vi "诊断标定3 - 副本.vi"(8 "CAN端口":u16(ring), 9 "设备索引号":u16(ring), 10 "CAN卡类型":u32(ring)=21) -> ()   [LabVIEW 2013] (continued)
                n3216 = Index Array(array=w4254, index=w4244) -> (element=w4249:dbl)
                n3217 = Index Array(array=w4248, index=w4244) -> (element=w4246:string)
                n3218 = Index Array(array=w4251, index=w4244) -> (element=w4247:u32)
                n3219 = stacked-sequence {
                  seq-local: [_ _ _ w4278 _ _] -> [_ _ _ _ w4287 _]
                  tunnel: w4250 -> [_ _ w4266 _ _ _]
                  tunnel: w4249 -> [_ _ w4265 _ _ _]
                  tunnel: w4253 -> [_ _ w4260 _ _ _]
                  tunnel: w4252 -> [_ _ w4263 _ _ _]
                  tunnel: w4247 -> [_ _ w4261 _ _ _]
                  tunnel: w4246 -> [_ _ w4259 _ w4286 _]
                  tunnel: w4245 -> [_ _ _ _ _ w4299]
                  tunnel: w4244 -> [_ _ _ _ _ w4298]
                  tunnel: w4243 -> [_ _ _ _ _ w4296]
                  frame #0 {
                    w4257 = FALSE ("流控帧")
                    w4256 = TRUE ("流控帧 2")
                    n3220 = call <vilib>:"Set Busy.vi"("disable click? (T)"=w4257) -> ()  [unwired: 3 in, 8 out]
                    n3221 = global write "EV05全局变量1.vi" "读取超时"(w4257) -> ()
                    n3222 = global write "EV05全局变量1.vi" "流控帧"(w4257) -> ()
                    n3223 = local write "消除"(w4256) -> ()
                    n3224 = local write "控制1"(w4256) -> ()
                    n3225 = global write "EV05全局变量1.vi" "流控帧 2"(w4256) -> ()
                    n3226 = local write "写?"(w4256) -> ()
                  }
                  frame #1 {
                    n3227 = Wait Until Next ms Multiple(millisecond multiple=u32 50 ("毫秒倍数")) -> ()  [unwired: 1 out]
                  }
                  frame #2 {
                    n3228 = global write "全局 1.vi" "名称"(w4259) -> ()
                    n3229 = local write "命令序号"(w4261) -> ()
                    n3230 = local write "命令"(w4260) -> ()
                    n3231 = local read "设备索引号"() -> (w4268:u16)
                    n3232 = local read "CAN卡类型"() -> (w4269:u32)
                    n3233 = Increment(x=w4265) -> (x+1=w4262:dbl)
                    n3234 = local read "CAN端口"() -> (w4267:u16)
                    n3235 = Reshape Array(w4266, w4262) -> (w4264:dbl[])
                    n3236 = stacked-sequence {
                      tunnel: w4269 -> [_ w4277]
                      tunnel: w4268 -> [_ w4276]
                      tunnel: w4267 -> [_ w4275]
                      tunnel: w4264 -> [_ w4274]
                      tunnel: w4263 -> [_ w4273]
                      tunnel: w4261 -> [_ w4272]
                      tunnel: w4260 -> [_ w4271]
                      frame #0 {
                      }
                      frame #1 {
                        n3237 = call "多帧发送机制(EV05).vi"("can卡类型"=w4277, "设备索引号"=w4276, "CAN端口"=w4275, "命令"=w4271, "板号"=w4273, "命令序号"=w4272, "输入数据"=w4274) -> ("错误输出"=w4270:errorcluster)  [unwired: 1 in, 11 out]
                        n3238 = call <vilib>:"Clear Errors.vi"("error in (no error)"=w4270) -> ()  [unwired: 6 in, 1 out]
                      }
                    }
                  }
                  frame #3 {
                    n3239 = while {
                      tunnel: [w4280] -> w4278
                      i -> [w4285]
                      stop <- w4282 stop-if-true
                      n3240 = local read "强制终止读写标记"() -> (w4279:bool)
                      n3241 = global read "EV05全局变量1.vi" "读取超时"() -> (w4280:bool)
                      n3242 = Greater Or Equal?(x=w4285, y=30) -> (x >= y?=w4283:bool)
                      n3243 = Wait Until Next ms Multiple(millisecond multiple=u32 100 ("毫秒倍数")) -> ()  [unwired: 1 out]
                      n3244 = Compound Arithmetic op=OR(w4279, w4280, w4283) -> (w4282:bool)
                    }
                  }
                  frame #4 {
                    n3245 = call <vilib>:"Unset Busy.vi"() -> ()  [unwired: 2 in, 10 out]
                    n3246 = case shown="假" w4287 {
                      tunnel: w4286 -> [w4288 _]
                      frame False {
                        n3247 = control-ref of="结果"() -> (w4292:refnum<vi>)
                        n3248 = Concatenate Strings(w4288, "       写入失败" ("字符串")) -> (w4291:string)
                        n3249 = Build Array(w4291) -> (w4290:string[])
                        n3250 = call "表格编辑.vi"("新元素/子数组"=w4290, "活动单元格:单元格背景色"=u32 16740749, "MCListbox引用句柄"=w4292) -> ()  [unwired: 9 out]
                      }
                      frame True {
                      }
                    }
                  }
                  frame #5 {
                    n3251 = Increment(x=w4298) -> (x+1=w4294:i32)
                    n3252 = Equal?(x=w4299, y=w4294) -> (x = y?=w4297:bool)
                    n3253 = And(x=w4296, y=w4297) -> (x .and. y?=w4295:bool)
                    n3254 = case shown="真" w4295 {
                      frame False {
                      }
                      frame True {
                        n3255 = control-ref of="结果"() -> (w4303:refnum<vi>)
                        n3256 = Concatenate Strings("写入完成" ("字符串")) -> (w4302:string)
                        n3257 = Build Array(w4302) -> (w4301:string[])
                        n3258 = call "表格编辑.vi"("新元素/子数组"=w4301, "活动单元格:单元格背景色"=u32 21937, "MCListbox引用句柄"=w4303) -> ()  [unwired: 9 out]
                      }
                    }
                  }
                }
              }
              n3259 = local read "强制终止读写标记"() -> (w4196:bool)
              n3260 = Or(x=w4194, y=w4196) -> (x .or. y?=w4195:bool)
            }
            n3261 = stacked-sequence {
              tunnel: w4186 -> [_]
              frame #0 {
                n3262 = call <vilib>:"Unset Busy.vi"() -> ()  [unwired: 2 in, 10 out]
                n3263 = local write "强制终止读写标记"(FALSE ("强制停止")) -> ()
              }
            }
          }
          frame "单个读取" {
            n3264 = stacked-sequence {
              tunnel: [w4336] -> w4334
              frame #0 {
                n3265 = local read "主从选择"() -> (w4337:enum32{"主板", "从板"})
                n3266 = case shown="\"主板\", 默认" w4337 {
                  tunnel: [w4350 w4433] -> w4339
                  tunnel: [w4349 w4434] -> w4344
                  tunnel: [0 ("从板号") w4430] -> w4343
                  tunnel: [0 ("板号") u8 0 ("板号")] -> w4342
                  tunnel: [w4345 w4429] -> w4340
                  frame "主板", Default {
                    n3267 = local read "主板选项"() -> (w4346:string)
                    n3268 = case shown="\"二维码\"" w4346 {
                      tunnel: [_ u8[] [1, 2, 3, 4, 5, 6, 13, 8, 7, 9, 10, 11, 12] u8[] [1] u8[] [1] u8[] [1] u8[] [2] u8[] [3] u8[] [4] u8[] [5] u8[] [6] u8[] [13] u8[] [7] u8[] [8] u8[] [9] u8[] [10] u8[] [14] u8[] [11] u8[] [12] u8[] [2] u8[] [3] u8[] [1] u8[] [2] u8[] [1] u8[] [2] u8[] [3] u8[] [4] u8[] [1, 2, 3, 4]] -> w4350
                      tunnel: [_ u8 128 ("命令") u8 129 ("命令") u8 128 ("命令") u8 140 ("命令") u8 128 ("命令") u8 128 ("命令") u8 128 ("命令") u8 128 ("命令") u8 128 ("命令") u8 128 ("命令") u8 128 ("命令") u8 128 ("命令") u8 128 ("命令") u8 128 ("命令") u8 128 ("命令") u8 128 ("命令") u8 128 ("命令") u8 129 ("命令") u8 129 ("命令") u8 130 ("命令") u8 130 ("命令") u8 132 ("命令") u8 132 ("命令") u8 132 ("命令") u8 132 ("命令") u8 132 ("命令")] -> w4349
                      tunnel: [_ string[] ["产品编号", "电压个数", "通道电压数", "电压起始值", "温度个数", "温度起始值", "保险位置", "电池额定实际容量", "SOC", "配置文件版本", "参数修改记录", "车牌号", "SOH"] string[] ["一级故障阀值"] string[] ["产品编号"] string[] ["读二维码"] string[] ["电压个数"] string[] ["通道电压数"] string[] ["电压起始值"] string[] ["温度个数"] string[] ["温度起始值"] string[] ["保险位置"] string[] ["SOC"] string[] ["电池额定实际容量"] string[] ["配置文件版本"] string[] ["参数修改记录"] string[] ["校正时钟"] string[] ["车牌号"] string[] ["SOH"] string[] ["二级故障阀值"] string[] ["三级故障阀值"] string[] ["加热控制参数"] string[] ["充电控制参数"] string[] ["电池信息1"] string[] ["电池包组号"] string[] ["充放电安时"] string[] ["电池充放电次数"] string[] ["电池信息1", "电池包组号", "充放电安时", "电池充放电次数"]] -> w4345
                      frame "假", Default {
                      }
                      frame "项目信息" {
                      }
                      frame "SOC过低", "SOC过高", "SOH过低", "充电电流过高", "单体电压过低", "单体电压过高", "单组电压不均衡", "单组温度不均衡", "放电电流过高", "极柱温度过高", "内阻过大", "温度过低", "温度过高", "一级故障阀值", "整组电压不均衡", "整组温度不均衡", "总电压过低", "总电压过高" {
                      }
                      frame "产品编号" {
                      }
                      frame "二维码" {
                      }
                      frame "电压个数" {
                      }
                      frame "通道电压数" {
                      }
                      frame "电压起始值" {
                      }
                      frame "温度个数" {
                      }
                      frame "温度起始值" {
                      }
                      frame "保险位置" {
                      }
                      frame "SOC" {
                      }
                      frame "电池额定实际容量" {
                      }
                      frame "配置文件版本" {
                      }
                      frame "参数修改记录" {
                      }
                      frame "校正时钟" {
                      }
                      frame "车牌号" {
                      }
                      frame "SOH" {
                      }
                      frame "SOC过低(2)", "SOC过高(2)", "SOH过低(2)", "充电电流过高(2)", "单体电压过低(2)", "单体电压过高(2)", "单组电压不均衡(2)", "单组温度不均衡(2)", "二级故障阀值", "放电电流过高(2)", "极柱温度过高(2)", "内阻过大(2)", "温度过低(2)", "温度过高(2)", "整组电压不均衡(2)", "整组温度不均衡(2)", "总电压过低(2)", "总电压过高(2)" {
                      }
                      frame "SOC过低(3)", "SOC过高(3)", "SOH过低(3)", "充电电流过高(3)", "单体电压过低(3)", "单体电压过高(3)", "单组电压不均衡(3)", "单组温度不均衡(3)", "放电电流过高(3)", "极柱温度过高(3)", "内阻过大(3)", "三级故障阀值", "温度过低(3)", "温度过高(3)", "整组电压不均衡(3)", "整组温度不均衡(3)", "总电压过低(3)", "总电压过高(3)" {
                      }
                      frame "风机关闭温差", "风机关闭温度", "风机开启温差", "风机开启温度", "加热关闭温差", "加热关闭温度", "加热开启温度", "加热控制参数" {
                      }
                      frame "充电控制参数", "电流步长", "最大允许充电电流", "最大允许充电温度", "最大允许单体电压", "最大允许总电压", "最小允许充电电流", "最小允许充电温度", "最小允许单体电压" {
                      }
                      frame "电池信息1" {
                      }
                      frame "电池包组号" {
                      }
                      frame "充放电安时" {
                      }
                      frame "电池充放电次数" {
                      }
                      frame "电池信息" {
                      }
                    }
                  }
                  frame "从板" {
                    n3269 = local read "从板选项"() -> (w4431:string)
                    n3270 = case shown="\"二维码\"" w4431 {
                      tunnel: [_ u8 0 ("命令") u8 10 ("命令") u8 0 ("命令") u8 0 ("命令") u8 0 ("命令") u8 0 ("命令") u8 0 ("命令") u8 0 ("命令") u8 2 ("命令") u8 2 ("命令") u8 2 ("命令") u8 3 ("命令") u8 6 ("命令") u8 6 ("命令") u8 6 ("命令") u8 3 ("命令") u8 3 ("命令") u8 3 ("命令") u8 3 ("命令") u8 3 ("命令") u8 3 ("命令") u8 3 ("命令")] -> w4434
                      tunnel: [_ u8[] [6] u8[] [1] u8[] [6, 1, 2, 3, 4, 5] u8[] [1] u8[] [2] u8[] [3] u8[] [4] u8[] [5] u8[] [1] u8[] [2] u8[] [3] u8[] [1, 2, 3, 4, 5, 6, 7] u8[] [1, 2] u8[] [2] u8[] [1] u8[] [1] u8[] [2] u8[] [3] u8[] [4] u8[] [5] u8[] [6] u8[] [7]] -> w4433
                      tunnel: [_ string[] ["从板号"] string[] ["读二维码"] string[] ["从板号", "电压起始值", "通道电压个数", "保险位置", "温度起始值", "加热控制参数"] string[] ["电压起始值"] string[] ["通道电压节数"] string[] ["保险位置"] string[] ["温度起始值"] string[] ["加热控制参数"] string[] ["一级故障阀值"] string[] ["二级故障阀值"] string[] ["三级故障阀值"] string[] ["电池包信息1", "电池包序号", "充放电安时", "充电次数时间", "SOC", "车牌号", "充电参数"] string[] ["均衡阀值", "充电结束电压"] string[] ["充电结束电压"] string[] ["均衡阀值"] string[] ["电池包信息1"] string[] ["电池包序号"] string[] ["充放电安时"] string[] ["充电次数时间"] string[] ["SOC"] string[] ["车牌号"] string[] ["充电参数"]] -> w4429
                      frame "假", Default {
                      }
                      frame "从板号" {
                      }
                      frame "二维码" {
                      }
                      frame "从板信息" {
                      }
                      frame "电压个数" {
                      }
                      frame "通道电压节数" {
                      }
                      frame "保险位置" {
                      }
                      frame "温度个数" {
                      }
                      frame "风机关闭温差", "风机关闭温度", "风机开启温差", "风机开启温度", "加热关闭温差", "加热关闭温度", "加热开启温度", "加热控制参数" {
                      }
                      frame "SOC过低", "电压不均衡", "电压过低", "电压过高", "温度不均衡", "温度过低", "温度过高", "一级故障阀值" {
                      }
                      frame "SOC过低(2)", "电压不均衡(2)", "电压过低(2)", "电压过高(2)", "二级故障阀值", "温度不均衡(2)", "温度过低(2)", "温度过高(2)" {
                      }
                      frame "SOC过低(3)", "电压不均衡(3)", "电压过低(3)", "电压过高(3)", "三级故障阀值", "温度不均衡(3)", "温度过低(3)", "温度过高(3)" {
                      }
                      frame "快换参数" {
                      }
                      frame "均衡参数" {
                      }
                      frame "充电结束电压" {
                      }
                      frame "均衡阀值" {
                      }
                      frame "电池包信息1" {
                      }
                      frame "电池包序号" {
                      }
                      frame "充放电安时" {
                      }
                      frame "充电次数时间" {
                      }
                      frame "SOC" {
                      }
                      frame "车牌号" {
                      }
                      frame "充电参数" {
                      }
                    }
                    n3271 = local read "从板号"() -> (w4430:u8)
                  }
                }
                n3272 = Build Array(w4342) -> (w4341:i32[])
                n3273 = local write "命令"(w4344) -> ()
                n3274 = Array Size(array=w4339) -> (size(s)=w4338:i32)
                n3275 = for {
                  tunnel: w4339 -> [w4509] mode=indexing
                  tunnel: w4344 -> [w4508]
                  tunnel: w4343 -> [w4507]
                  tunnel: w4341 -> [w4506]
                  tunnel: w4340 -> [w4505] mode=indexing
                  tunnel: w4338 -> [w4504]
                  tunnel: w4337 -> [w4502]
                  tunnel: [w4501] -> w4336
                  i -> [w4503]
                  n3276 = while {
                    tunnel: w4509 -> [w4518]
                    tunnel: w4508 -> [w4517]
                    tunnel: w4507 -> [w4516]
                    tunnel: w4506 -> [w4515]
                    tunnel: w4505 -> [w4514]
                    tunnel: w4504 -> [w4513]
                    tunnel: w4503 -> [w4512]
                    tunnel: w4502 -> [w4511]
                    tunnel: [w4510] -> w4501
                    stop <- w4510 stop-if-true
                    n3277 = stacked-sequence {
                      seq-local: [_ _ _ _ w4668 _ _] -> [_ _ _ _ _ w4677 _]
                      tunnel: w4518 -> [_ _ _ w4656 _ _ _]
                      tunnel: w4517 -> [_ _ _ w4655 _ _ _]
                      tunnel: w4516 -> [_ _ _ w4654 _ _ _]
                      tunnel: w4515 -> [_ _ _ w4653 _ _ _]
                      tunnel: [_ _ _ _ w4669 _ _] -> w4510
                      tunnel: w4514 -> [w4520 _ _ _ _ w4678 _]
                      tunnel: w4513 -> [_ _ _ _ _ _ w4688]
                      tunnel: w4512 -> [_ _ _ _ _ _ w4687]
                      tunnel: w4511 -> [w4519 _ _ _ _ _ _]
                      frame #0 {
                        n3278 = case shown="\"从板\"" w4519 {
                          tunnel: w4520 -> [w4521 w4613]
                          frame "主板", Default {
                            n3279 = case shown="\"读二维码\"" w4521 {
                              frame "假", Default {
                              }
                              frame "产品编号" {
                                n3280 = control-ref of="产品编号"() -> (w4523:refnum<vi>)
                                n3281 = property class="Str"(reference=w4523, "Value"="") -> ()  [unwired: 1 in, 2 out]
                              }
                              frame "读二维码" {
                                n3282 = local write "二维码信息"("" ("二维码信息")) -> ()
                              }
                              frame "电压个数" {
                                n3283 = local read "从板个数"() -> (w4525:dbl)
                                n3284 = control-ref of="项目信息"() -> (w4529:refnum<vi>)
                                n3285 = for {
                                N: w4525 -> [_]
                                tunnel: [""] -> w4528 mode=indexing
                                }
                                n3286 = call "表格数据输入-8.6.vi"("行数"=u32 0, "列数"=u32 1, "字符串数组"=w4528, "表格引用"=w4529) -> ()  [unwired: 8 in]
                              }
                              frame "通道电压数" {
                                n3287 = control-ref of="项目信息"() -> (w4535:refnum<vi>)
                                n3288 = for {
                                N: 20 -> [_]
                                tunnel: [""] -> w4534 mode=indexing
                                }
                                n3289 = local read "从板个数"() -> (w4536:dbl)
                                n3290 = Increment(x=w4536) -> (x+1=w4532:dbl)
                                n3291 = call "表格数据输入-8.6.vi"("行数"=w4532, "列数"=u32 1, "字符串数组"=w4534, "表格引用"=w4535) -> ()  [unwired: 8 in]
                              }
                              frame "电压起始值" {
                                n3292 = local read "从板个数"() -> (w4540:dbl)
                                n3293 = Increment(x=w4540) -> (x+1=w4539:dbl)
                                n3294 = control-ref of="项目信息"() -> (w4546:refnum<vi>)
                                n3295 = for {
                                N: w4539 -> [_]
                                tunnel: [""] -> w4545 mode=indexing
                                }
                                n3296 = Multiply(x=u8 1, y=w4540) -> (x*y=w4542:dbl)
                                n3297 = Add(x=w4542, y=u8 21) -> (x+y=w4538:dbl)
                                n3298 = call "表格数据输入-8.6.vi"("行数"=w4538, "列数"=u32 1, "字符串数组"=w4545, "表格引用"=w4546) -> ()  [unwired: 8 in]
                              }
                              frame "温度个数" {
                                n3299 = local read "从板个数"() -> (w4550:dbl)
                                n3300 = Increment(x=w4550) -> (x+1=w4549:dbl)
                                n3301 = control-ref of="项目信息"() -> (w4556:refnum<vi>)
                                n3302 = for {
                                N: w4549 -> [_]
                                tunnel: [""] -> w4555 mode=indexing
                                }
                                n3303 = Multiply(x=u8 2, y=w4550) -> (x*y=w4552:dbl)
                                n3304 = Add(x=w4552, y=u8 22) -> (x+y=w4548:dbl)
                                n3305 = call "表格数据输入-8.6.vi"("行数"=w4548, "列数"=u32 1, "字符串数组"=w4555, "表格引用"=w4556) -> ()  [unwired: 8 in]
                              }
                              frame "温度起始值" {
                                n3306 = local read "从板个数"() -> (w4560:dbl)
                                n3307 = Increment(x=w4560) -> (x+1=w4559:dbl)
                                n3308 = control-ref of="项目信息"() -> (w4566:refnum<vi>)
                                n3309 = for {
                                N: w4559 -> [_]
                                tunnel: [""] -> w4565 mode=indexing
                                }
                                n3310 = Multiply(x=u8 3, y=w4560) -> (x*y=w4562:dbl)
                                n3311 = Add(x=w4562, y=u8 23) -> (x+y=w4558:dbl)
                                n3312 = call "表格数据输入-8.6.vi"("行数"=w4558, "列数"=u32 1, "字符串数组"=w4565, "表格引用"=w4566) -> ()  [unwired: 8 in]
                              }
                              frame "保险位置" {
                                n3313 = local read "从板个数"() -> (w4570:dbl)
                                n3314 = control-ref of="项目信息"() -> (w4576:refnum<vi>)
                                n3315 = for {
                                N: 10 -> [_]
                                tunnel: [""] -> w4575 mode=indexing
                                }
                                n3316 = Multiply(x=u8 4, y=w4570) -> (x*y=w4572:dbl)
                                n3317 = Add(x=w4572, y=u8 24) -> (x+y=w4569:dbl)
                                n3318 = call "表格数据输入-8.6.vi"("行数"=w4569, "列数"=u32 1, "字符串数组"=w4575, "表格引用"=w4576) -> ()  [unwired: 8 in]
                              }
                              frame "电池额定实际容量" {
                                w4578 = 0.0 ("值")
                                n3319 = control-ref of="电池实际容量(A)"() -> (w4579:refnum<vi>)
                                n3320 = control-ref of="电池额定容量(A)"() -> (w4580:refnum<vi>)
                                n3321 = property class="DigNum (严格)"(reference=w4579, "Value"=w4578) -> ()  [unwired: 1 in, 2 out]
                                n3322 = property class="DigNum (严格)"(reference=w4580, "Value"=w4578) -> ()  [unwired: 1 in, 2 out]
                              }
                              frame "SOC" {
                                n3323 = control-ref of="SOC(%)"() -> (w4581:refnum<vi>)
                                n3324 = property class="DigNum (严格)"(reference=w4581, "Value"=0.0 ("值")) -> ()  [unwired: 1 in, 2 out]
                              }
                              frame "配置文件版本" {
                                n3325 = control-ref of="配置文件版本"() -> (w4583:refnum<vi>)
                                n3326 = property class="Str"(reference=w4583, "Value"="" ("值")) -> ()  [unwired: 1 in, 2 out]
                              }
                              frame "参数修改记录" {
                                n3327 = control-ref of="使用者"() -> (w4586:refnum<vi>)
                                n3328 = control-ref of="系统时钟"() -> (w4587:refnum<vi>)
                                n3329 = property class="DigNum (严格)"(reference=w4586, "Value"=0.0 ("值")) -> ()  [unwired: 1 in, 2 out]
                                n3330 = property class="Str"(reference=w4587, "Value"="" ("值")) -> ()  [unwired: 1 in, 2 out]
                              }
                              frame "校正时钟" {
                                n3331 = control-ref of="系统时钟"() -> (w4589:refnum<vi>)
                                n3332 = property class="Str"(reference=w4589, "Value"="" ("值")) -> ()  [unwired: 1 in, 2 out]
                              }
                              frame "车牌号" {
                                n3333 = control-ref of="车架(牌)号"() -> (w4591:refnum<vi>)
                                n3334 = property class="Str"(reference=w4591, "Value"="" ("值")) -> ()  [unwired: 1 in, 2 out]
                              }
                              frame "SOH" {
                                n3335 = control-ref of="SOH(%)"() -> (w4594:refnum<vi>)
                                n3336 = property class="DigNum (严格)"(reference=w4594, "Value"=0.0 ("值")) -> ()  [unwired: 1 in, 2 out]
                              }
                              frame "一级故障阀值" {
                                n3337 = local write "一级故障"(T10 {"总电压过高"=0.0, "整组电压不均衡"=0.0, "SOC过高"=0.0, "单体电压过高"=0.0, "总电压过低"=0.0, "温度过高"=0.0, "温度过低"=0.0, "单组电压不均衡"=0.0, "整组温度不均衡"=0.0, "单组温度不均衡"=0.0, "单体电压过低"=0.0, "充电电流过高"=0.0, "放电电流过高"=0.0, "SOC过低"=0.0, "内阻过大"=0.0, "极柱温度过高"=0.0, "SOH过低"=0.0} ("一级故障")) -> ()
                              }
                              frame "二级故障阀值" {
                                n3338 = local write "一级故障 2"(T10 {"总电压过高"=0.0, "整组电压不均衡"=0.0, "SOC过高"=0.0, "单体电压过高"=0.0, "总电压过低"=0.0, "温度过高"=0.0, "温度过低"=0.0, "单组电压不均衡"=0.0, "整组温度不均衡"=0.0, "单组温度不均衡"=0.0, "单体电压过低"=0.0, "充电电流过高"=0.0, "放电电流过高"=0.0, "SOC过低"=0.0, "内阻过大"=0.0, "极柱温度过高"=0.0, "SOH过低"=0.0} ("一级故障")) -> ()
                              }
                              frame "三级故障阀值" {
                                n3339 = local write "一级故障 3"(T10 {"总电压过高"=0.0, "整组电压不均衡"=0.0, "SOC过高"=0.0, "单体电压过高"=0.0, "总电压过低"=0.0, "温度过高"=0.0, "温度过低"=0.0, "单组电压不均衡"=0.0, "整组温度不均衡"=0.0, "单组温度不均衡"=0.0, "单体电压过低"=0.0, "充电电流过高"=0.0, "放电电流过高"=0.0, "SOC过低"=0.0, "内阻过大"=0.0, "极柱温度过高"=0.0, "SOH过低"=0.0} ("一级故障")) -> ()
                              }
                              frame "加热控制参数" {
                                n3340 = local write "加热控制参数"(T11 {"风机开启温度"=0.0, "风机关闭温度"=0.0, "加热开启温度"=0.0, "加热关闭温度"=0.0, "风机开启温差"=0.0, "风机关闭温差"=0.0, "加热关闭温差"=0.0} ("加热控制参数")) -> ()
                              }
                              frame "充电控制参数" {
                                n3341 = local write "一级故障 5"(T12 {"最大允许单体电压"=0.0, "最大允许总电压"=0.0, "最小允许单体电压"=0.0, "最大允许充电电流"=0.0, "最小允许充电电流"=0.0, "最大允许充电温度"=0.0, "最小允许充电温度"=0.0, "电流步长"=0.0} ("一级故障 5")) -> ()
                              }
                              frame "电池信息1" {
                                w4600 = ""
                                w4601 = 0.0 ("电池串联")
                                n3342 = local read "电池信息"() -> (w4603:T13)
                                n3343 = Bundle By Name(cluster=w4603, "电池串联"=w4601, "电池并联"=w4601, "电池包额定容量"=w4601, "电池包额定能量(kWh)"=w4601, "电池包额定总电压"=w4601, "实际容量"=w4601, "电池厂家"=w4600, "电池类型"=w4600, "电池生产日期"=w4600) -> (w4602:T13)
                                n3344 = local write "电池信息"(w4602) -> ()
                              }
                              frame "电池包组号" {
                                n3345 = local read "电池信息"() -> (w4606:T13)
                                n3346 = Bundle By Name(cluster=w4606, "电池包组号"="") -> (w4605:T13)
                                n3347 = local write "电池信息"(w4605) -> ()
                              }
                              frame "充放电安时" {
                                w4607 = 0.0 ("累计充电总安时")
                                n3348 = local read "电池信息"() -> (w4609:T13)
                                n3349 = Bundle By Name(cluster=w4609, "累计充电总安时"=w4607, "累计放电总安时"=w4607) -> (w4608:T13)
                                n3350 = local write "电池信息"(w4608) -> ()
                              }
                              frame "电池充放电次数" {
                                w4610 = 0.0 ("累计充电总安时")
                                n3351 = local read "电池信息"() -> (w4612:T13)
                                n3352 = Bundle By Name(cluster=w4612, "电池充满次数"=w4610, "电池放空次数"=w4610, "电池充电次数"=w4610) -> (w4611:T13)
                                n3353 = local write "电池信息"(w4611) -> ()
                              }
                            }
                          }
                          frame "从板" {
                            n3354 = case shown="\"读二维码\"" w4613 {
                              frame "假", Default {
                              }
                              frame "电压起始值" {
                                n3355 = control-ref of="项目信息 2"() -> (w4615:refnum<vi>)
                                n3356 = for {
                                N: 1 -> [_]
                                tunnel: [""] -> w4618 mode=indexing
                                }
                                n3357 = call "表格数据输入-8.6.vi"("行数"=u32 0, "列数"=u32 1, "字符串数组"=w4618, "表格引用"=w4615) -> ()  [unwired: 8 in]
                              }
                              frame "读二维码" {
                                n3358 = local write "二维码信息 2"("" ("二维码信息 2")) -> ()
                              }
                              frame "通道电压节数" {
                                n3359 = control-ref of="项目信息 2"() -> (w4621:refnum<vi>)
                                n3360 = for {
                                N: 5 -> [_]
                                tunnel: [""] -> w4625 mode=indexing
                                }
                                n3361 = call "表格数据输入-8.6.vi"("行数"=u32 22, "列数"=u32 1, "字符串数组"=w4625, "表格引用"=w4621) -> ()  [unwired: 8 in]
                              }
                              frame "保险位置" {
                                n3362 = control-ref of="项目信息 2"() -> (w4627:refnum<vi>)
                                n3363 = for {
                                N: 20 -> [_]
                                tunnel: [""] -> w4631 mode=indexing
                                }
                                n3364 = call "表格数据输入-8.6.vi"("行数"=u32 2, "列数"=u32 1, "字符串数组"=w4631, "表格引用"=w4627) -> ()  [unwired: 8 in]
                              }
                              frame "温度起始值" {
                                n3365 = control-ref of="项目信息 2"() -> (w4633:refnum<vi>)
                                n3366 = for {
                                N: 1 -> [_]
                                tunnel: [""] -> w4637 mode=indexing
                                }
                                n3367 = call "表格数据输入-8.6.vi"("行数"=u32 1, "列数"=u32 1, "字符串数组"=w4637, "表格引用"=w4633) -> ()  [unwired: 8 in]
                              }
                              frame "加热控制参数" {
                                n3368 = local write "加热控制参数"(T11 {"风机开启温度"=0.0, "风机关闭温度"=0.0, "加热开启温度"=0.0, "加热关闭温度"=0.0, "风机开启温差"=0.0, "风机关闭温差"=0.0, "加热关闭温差"=0.0} ("加热控制参数")) -> ()
                              }
                              frame "一级故障阀值" {
                                n3369 = local write "一级故障 6"(T15 {"电压过高"=0.0, "电压过低"=0.0, "温度过高"=0.0, "温度过低"=0.0, "电压不均衡(V)"=0.0, "温度不均衡"=0.0, "SOC过低"=0.0} ("一级故障 6")) -> ()
                              }
                              frame "二级故障阀值" {
                                n3370 = local write "一级故障 7"(T15 {"电压过高"=0.0, "电压过低"=0.0, "温度过高"=0.0, "温度过低"=0.0, "电压不均衡(V)"=0.0, "温度不均衡"=0.0, "SOC过低"=0.0} ("一级故障 7")) -> ()
                              }
                              frame "三级故障阀值" {
                                n3371 = local write "一级故障 8"(T15 {"电压过高"=0.0, "电压过低"=0.0, "温度过高"=0.0, "温度过低"=0.0, "电压不均衡(V)"=0.0, "温度不均衡"=0.0, "SOC过低"=0.0} ("一级故障 7")) -> ()
                              }
                              frame "均衡参数" {
                                n3372 = local write "均衡参数"(T17 {"充电结束电压(90%)"=0.0, "充电结束电压(91%)"=0.0, "充电结束电压(92%)"=0.0, "充电结束电压(93%)"=0.0, "充电结束电压(94%)"=0.0, "均衡计算-电压高阀值1级"=0.0, "均衡计算-电压高阀值2级"=0.0, "均衡计算-电压低阀值1级"=0.0, "均衡计算-电压低阀值2级"=0.0, "均衡计算-最低电压阀值"=0.0, "均衡停止-最低电压阀值"=0.0, "均衡计算-电压极差阀值"=0.0, "充电结束电压(95%)"=0.0, "充电结束电压(96%)"=0.0, "充电结束电压(97%)"=0.0, "充电结束电压(98%)"=0.0, "充电结束电压(99%)"=0.0, "充电结束电压(100%)"=0.0} ("均衡参数")) -> ()
                              }
                              frame "均衡阀值" {
                                w4644 = sgl 0.0 ("均衡计算-电压高阀值1级")
                                n3373 = local read "均衡参数"() -> (w4645:T17)
                                n3374 = Bundle By Name(cluster=w4645, "均衡计算-电压高阀值1级"=w4644, "均衡计算-电压高阀值2级"=w4644, "均衡计算-电压低阀值1级"=w4644, "均衡计算-电压低阀值2级"=w4644, "均衡计算-最低电压阀值"=w4644, "均衡停止-最低电压阀值"=w4644, "均衡计算-电压极差阀值"=w4644) -> (w4646:T17)
                                n3375 = local write "均衡参数"(w4646) -> ()
                              }
                              frame "充电结束电压" {
                                w4647 = sgl 0.0 ("均衡计算-电压高阀值1级")
                                n3376 = local read "均衡参数"() -> (w4648:T17)
                                n3377 = Bundle By Name(cluster=w4648, "充电结束电压(90%)"=w4647, "充电结束电压(91%)"=w4647, "充电结束电压(92%)"=w4647, "充电结束电压(93%)"=w4647, "充电结束电压(94%)"=w4647, "充电结束电压(95%)"=w4647, "充电结束电压(96%)"=w4647, "充电结束电压(97%)"=w4647, "充电结束电压(98%)"=w4647, "充电结束电压(99%)"=w4647, "充电结束电压(100%)"=w4647) -> (w4649:T17)
                                n3378 = local write "均衡参数"(w4649) -> ()
                              }
                            }
                          }
                        }
                      }
                      frame #1 {
                        w4650 = FALSE ("流控帧")
                        w4651 = TRUE ("流控帧 2")
                        n3379 = global write "EV05全局变量1.vi" "写入超时"(w4650) -> ()
                        n3380 = global write "EV05全局变量1.vi" "流控帧"(w4650) -> ()
                        n3381 = local write "写?"(w4650) -> ()
                        n3382 = call <vilib>:"Set Busy.vi"("disable click? (T)"=w4650) -> ()  [unwired: 3 in, 8 out]
                        n3383 = local write "消除"(w4651) -> ()
                        n3384 = local write "控制1"(w4651) -> ()
                        n3385 = global write "EV05全局变量1.vi" "流控帧 2"(w4651) -> ()
                      }
                      frame #2 {
                        n3386 = Wait Until Next ms Multiple(millisecond multiple=u32 150 ("毫秒倍数")) -> ()  [unwired: 1 out]
                      }
                      frame #3 {
                        n3387 = local read "设备索引号"() -> (w4658:u16)
                        n3388 = local read "CAN卡类型"() -> (w4659:u32)
                        n3389 = local read "CAN端口"() -> (w4657:u16)
                        n3390 = stacked-sequence {
                          tunnel: w4659 -> [_ w4667]
                          tunnel: w4658 -> [_ w4666]
                          tunnel: w4657 -> [_ w4665]
                          tunnel: w4656 -> [_ w4664]
                          tunnel: w4655 -> [_ w4663]
                          tunnel: w4654 -> [_ w4662]
                          tunnel: w4653 -> [_ w4661]
                          frame #0 {
                          }
                          frame #1 {
                            n3391 = call "多帧发送机制(EV05).vi"("can卡类型"=w4667, "设备索引号"=w4666, "CAN端口"=w4665, "命令"=w4663, "板号"=w4662, "命令序号"=w4664, "输入数据"=w4661) -> ("错误输出"=w4660:errorcluster)  [unwired: 1 in, 11 out]
                            n3392 = call <vilib>:"Clear Errors.vi"("error in (no error)"=w4660) -> ()  [unwired: 6 in, 1 out]
                          }
                        }
                        "命令序号" <- w4656
                      }
                      frame #4 {
                        n3393 = while {
                          tunnel: [w4672] -> w4669
                          tunnel: [w4671] -> w4668
                          i -> [w4675]
                          stop <- w4672 stop-if-true
                          n3394 = local read "强制终止读写标记"() -> (w4670:bool)
                          n3395 = global read "EV05全局变量1.vi" "写入超时"() -> (w4671:bool)
                          n3396 = Greater Or Equal?(x=w4675, y=30) -> (x >= y?=w4673:bool)
                          n3397 = Compound Arithmetic op=OR(w4670, w4671, w4673) -> (w4672:bool)
                          n3398 = Wait Until Next ms Multiple(millisecond multiple=u32 100 ("毫秒倍数")) -> ()  [unwired: 1 out]
                        }
                      }
                      frame #5 {
                        n3399 = case shown="假" w4677 {
                          tunnel: w4678 -> [w4681 _]
                          frame False {
                            n3400 = control-ref of="结果"() -> (w4680:refnum<vi>)
                            n3401 = Concatenate Strings(w4681, "     读取失败" ("字符串")) -> (w4683:string)
                            n3402 = Build Array(w4683) -> (w4679:string[])
                            n3403 = call "表格编辑.vi"("新元素/子数组"=w4679, "活动单元格:单元格背景色"=u32 16740749, "MCListbox引用句柄"=w4680) -> ()  [unwired: 9 out]
                          }
                          frame True {
                          }
                        }
                      }
                      frame #6 {
                        n3404 = Increment(x=w4687) -> (x+1=w4686:i32)
                        n3405 = Equal?(x=w4688, y=w4686) -> (x = y?=w4685:bool)
                        n3406 = case shown="真" w4685 {
                          frame False {
                          }
                          frame True {
                            n3407 = control-ref of="结果"() -> (w4690:refnum<vi>)
                            n3408 = Concatenate Strings("读取完成" ("字符串")) -> (w4692:string)
                            n3409 = Build Array(w4692) -> (w4689:string[])
                            n3410 = call "表格编辑.vi"("新元素/子数组"=w4689, "活动单元格:单元格背景色"=u32 21937, "MCListbox引用句柄"=w4690) -> ()  [unwired: 9 out]
                          }
                        }
                      }
                    }
                  }
                }
              }
            }
            n3411 = stacked-sequence {
              tunnel: w4334 -> [_]
              frame #0 {
                n3412 = call <vilib>:"Unset Busy.vi"() -> ()  [unwired: 11 in, 1 out]
                n3413 = local write "强制终止读写标记"(FALSE ("强制停止")) -> ()
              }
            }
          }
          frame "全部读取" {
            n3414 = stacked-sequence {
              seq-local: [w4698 _ _] -> [_ _ w5259]
              seq-local: [w4697 _ _] -> [_ _ w5258]
              tunnel: [_ w4889 _] -> w4695
              frame #0 {
                n3415 = local read "主从选择"() -> (w4698:enum32{"主板", "从板"})
                n3416 = local read "路径"() -> (w4699:path)
                n3417 = Empty String/Path?(string/path=w4699) -> (empty?=w4697:bool)
                n3418 = disable-structure shown="禁用" {
                  disable-tunnel: w4699 -> [w4702 _]
                  disable-tunnel: w4697 -> [w4701 _]
                  disable-tunnel: w4698 -> [w4700 _]
                  frame Disabled {
                    n3419 = case shown="假" w4701 {
                      tunnel: w4702 -> [w4706 _]
                      tunnel: w4700 -> [w4705 _]
                      frame False {
                        n3420 = control-ref of="结果"() -> (w4703:refnum<vi>)
                        n3421 = call-poly <vilib>:"Read From Spreadsheet File.vi"("file path (dialog if empty)"=w4706) -> ("all rows"=w4704:string[][])  [unwired: 3 in, 7 out]
                        n3422 = case shown="\"主板\", 默认" w4705 {
                          tunnel: w4704 -> [w4708 w4803]
                          tunnel: w4703 -> [w4707 w4802]
                          frame "主板", Default {
                            n3423 = stacked-sequence {
                              tunnel: w4708 -> [w4717 w4741 w4798]
                              tunnel: w4707 -> [w4714 _ w4769]
                              frame #0 {
                                n3424 = Index Array(array=w4717, index (col)=3 ("禁用的索引 (列)")) -> (element=w4731:string[])  [unwired: 1 in]
                                n3425 = Index Array(array=w4717, index (col)=1 ("禁用的索引 (列)")) -> (element=w4737:string[])  [unwired: 1 in]
                                n3426 = Delete From Array(array=w4731, length=4 ("长度"), index=0 ("索引")) -> (deleted portion=w4728:string[], array with subset deleted=w4722:string[])
                                n3427 = Delete From Array(array=w4737, length=1 ("长度"), index=0 ("索引")) -> (deleted portion=w4734:string[], array with subset deleted=w4711:string[])
                                n3428 = Build Array("正在读取主板配置文件...") -> (w4715:string[])
                                n3429 = Index Array(array=w4722) -> (element #1=w4721:string, element #2=w4720:string, element #3=w4719:string, element #4=w4718:string)  [unwired: 4 in]
                                n3430 = for {
                                tunnel: w4728 -> [w4740] mode=indexing
                                tunnel: [w4739] -> w4727 mode=indexing
                                n3431 = Fract/Exp String To Number(string=w4740) -> (number=w4739:dbl)  [unwired: 4 out]
                                }
                                n3432 = Index Array(array=w4734) -> (element=w4733:string)  [unwired: 1 in]
                                n3433 = global write "读配置文件全局.vi" "表格输入"(w4711) -> ()
                                n3434 = call "表格编辑.vi"("新元素/子数组"=w4715, "活动单元格:单元格背景色"=u32 6618880, "MCListbox引用句柄"=w4714) -> ()  [unwired: 9 out]
                                n3435 = Decimal String To Number(string=w4733) -> (number=w4712:i32)  [unwired: 1 in, 2 out]
                                n3436 = global read "读配置文件全局.vi" "项目信息"() -> (w4710:T27)
                                n3437 = Index Array(array=w4727) -> (element #1=w4726:dbl, element #2=w4725:dbl, element #3=w4724:dbl, element #4=w4723:dbl)  [unwired: 4 in]
                                n3438 = global write "读配置文件全局.vi" "从板个数"(w4712) -> ()
                                n3439 = Bundle(cluster=w4710, "电池额定容量"=w4726, "电池实际容量"=w4725, "车牌号"=w4721, "配置文件版本"=w4720, "SOH"=w4723, "SOC"=w4724, "产品编号"=w4719, "系统时钟"=w4718) -> (w4709:T27)  [unwired: 1 out]
                                n3440 = global write "读配置文件全局.vi" "项目信息"(w4709) -> ()
                              }
                              frame #1 {
                                n3441 = Index Array(array=w4741, index (col)=3 ("禁用的索引 (列)")) -> (element=w4759:string[])  [unwired: 1 in]
                                n3442 = Index Array(array=w4741, index (col)=5 ("禁用的索引 (列)")) -> (element=w4753:string[])  [unwired: 1 in]
                                n3443 = for {
                                tunnel: w4753 -> [w4766] mode=indexing
                                tunnel: [w4765] -> w4752 mode=indexing
                                n3444 = Fract/Exp String To Number(string=w4766) -> (number=w4765:dbl)  [unwired: 4 out]
                                }
                                n3445 = Delete From Array(array=w4759, length=17 ("长度"), index=8 ("索引")) -> (deleted portion=w4757:string[])  [unwired: 1 out]
                                n3446 = for {
                                tunnel: w4757 -> [w4768] mode=indexing
                                tunnel: [w4767] -> w4755 mode=indexing
                                n3447 = Fract/Exp String To Number(string=w4768) -> (number=w4767:dbl)  [unwired: 4 out]
                                }
                                n3448 = global write "读配置文件全局.vi" "二级故障"(w4752) -> ()
                                n3449 = global write "读配置文件全局.vi" "一级故障"(w4755) -> ()
                                n3450 = Index Array(array=w4741, index (col)=7 ("禁用的索引 (列)")) -> (element=w4750:string[])  [unwired: 1 in]
                                n3451 = Index Array(array=w4741, index (col)=9 ("禁用的索引 (列)")) -> (element=w4747:string[])  [unwired: 1 in]
                                n3452 = for {
                                tunnel: w4750 -> [w4764] mode=indexing
                                tunnel: [w4763] -> w4749 mode=indexing
                                n3453 = Fract/Exp String To Number(string=w4764) -> (number=w4763:dbl)  [unwired: 4 out]
                                }
                                n3454 = for {
                                tunnel: w4747 -> [w4762] mode=indexing
                                tunnel: [w4761] -> w4746 mode=indexing
                                n3455 = Fract/Exp String To Number(string=w4762) -> (number=w4761:dbl)  [unwired: 4 out]
                                }
                                n3456 = Delete From Array(array=w4746, length=6 ("长度"), index=0 ("索引")) -> (deleted portion=w4743:dbl[], array with subset deleted=w4742:dbl[])
                                n3457 = global write "读配置文件全局.vi" "三级故障"(w4749) -> ()
                                n3458 = global write "读配置文件全局.vi" "加热控制参数"(w4743) -> ()
                                n3459 = global write "读配置文件全局.vi" "充电控制参数"(w4742) -> ()
                              }
                              frame #2 {
                                n3460 = call <vilib>:"Unset Busy.vi"() -> ()  [unwired: 2 in, 10 out]
                                n3461 = Index Array(array=w4798, index (col)=11 ("禁用的索引 (列)")) -> (element=w4795:string[])  [unwired: 1 in]
                                n3462 = Delete From Array(array=w4795, length=6 ("长度"), index=0 ("索引")) -> (deleted portion=w4777:string[], array with subset deleted=w4776:string[])
                                n3463 = for {
                                tunnel: w4776 -> [w4801] mode=indexing
                                tunnel: [w4800] -> w4794 mode=indexing
                                n3464 = Fract/Exp String To Number(string=w4801) -> (number=w4800:dbl)  [unwired: 4 out]
                                }
                                n3465 = Index Array(array=w4777) -> (element #1=w4793:string, element #2=w4792:string, element #3=w4791:string, element #4=w4790:string, element #5=w4789:string, element #6=w4788:string)  [unwired: 6 in]
                                n3466 = Index Array(array=w4794) -> (element #1=w4787:dbl, element #2=w4786:dbl, element #3=w4785:dbl, element #4=w4784:dbl, element #5=w4783:dbl, element #6=w4782:dbl, element #7=w4781:dbl, element #8=w4780:dbl, element #9=w4779:dbl, element #10=w4778:dbl, element #11=w4773:dbl)  [unwired: 11 in]
                                n3467 = global read "读配置文件全局.vi" "电池信息"() -> (w4775:T28)
                                n3468 = Build Array("配置文件读取完成") -> (w4771:string[])
                                n3469 = Bundle(cluster=w4775, "电池串联"=w4787, "电池并联"=w4786, "累计放电总安时"=w4784, "电池包额定容量"=w4783, "电池包额定能量"=w4782, "电池包额定总电压"=w4781, "累计充电总安时"=w4785, "电池充满次数"=w4780, "电池放空次数"=w4779, "电池充电次数"=w4778, "电池生产日期"=w4793, "电池厂家"=w4792, "电池类型"=w4791, "电池包组号"=w4790, "电池包产权标识"=w4789, "电池应用车型"=w4788, "实际容量"=w4773) -> (w4774:T28)
                                n3470 = call "表格编辑.vi"("新元素/子数组"=w4771, "活动单元格:单元格背景色"=u32 6618880, "MCListbox引用句柄"=w4769) -> ()  [unwired: 9 out]
                                n3471 = global write "读配置文件全局.vi" "电池信息"(w4774) -> ()
                              }
                            }
                          }
                          frame "从板" {
                            n3472 = stacked-sequence {
                              tunnel: w4803 -> [w4811 w4839 w4883]
                              tunnel: w4802 -> [w4808 _ w4859]
                              frame #0 {
                                n3473 = Index Array(array=w4811, index (col)=1 ("禁用的索引 (列)")) -> (element=w4821:string[])  [unwired: 1 in]
                                n3474 = Index Array(array=w4811, index (col)=3 ("禁用的索引 (列)")) -> (element=w4815:string[])  [unwired: 1 in]
                                n3475 = Delete From Array(array=w4821, length=1 ("长度"), index=0 ("索引")) -> (deleted portion=w4818:string[], array with subset deleted=w4805:string[])
                                n3476 = Delete From Array(array=w4815, length=6 ("长度"), index=0 ("索引")) -> (deleted portion=w4812:string[])  [unwired: 1 out]
                                n3477 = for {
                                tunnel: w4812 -> [w4824] mode=indexing
                                tunnel: [w4823] -> w4804 mode=indexing
                                i -> [w4825]
                                n3478 = Fract/Exp String To Number(string=w4824, default (0 dbl)=w4825) -> (number=w4823:i32)  [unwired: 3 out]
                                }
                                n3479 = Index Array(array=w4818) -> (element=w4817:string)  [unwired: 1 in]
                                n3480 = global write "读配置文件全局2.vi" "表格"(w4805) -> ()
                                n3481 = Build Array("正在读取从板配置文件...") -> (w4809:string[])
                                n3482 = Decimal String To Number(string=w4817) -> (number=w4806:i32)  [unwired: 1 in, 2 out]
                                n3483 = call "表格编辑.vi"("新元素/子数组"=w4809, "活动单元格:单元格背景色"=u32 6618880, "MCListbox引用句柄"=w4808) -> ()  [unwired: 9 out]
                                n3484 = global write "读配置文件全局2.vi" "加热控制参数"(w4804) -> ()
                                n3485 = global write "读配置文件全局2.vi" "从板板号"(w4806) -> ()
                              }
                              frame #1 {
                                n3486 = Index Array(array=w4839, index (col)=3 ("禁用的索引 (列)")) -> (element=w4829:string[])  [unwired: 1 in]
                                n3487 = Array Subset(array=w4829, index=6 ("索引"), length=7 ("长度")) -> (w4836:string[])
                                n3488 = Array Subset(array=w4829, index=13 ("索引"), length=7 ("长度")) -> (w4835:string[])
                                n3489 = Array Subset(array=w4829, index=20 ("索引"), length=7 ("长度")) -> (w4830:string[])
                                n3490 = for {
                                tunnel: w4836 -> [w4846] mode=indexing
                                tunnel: [w4845] -> w4826 mode=indexing
                                n3491 = Fract/Exp String To Number(string=w4846) -> (number=w4845:dbl)  [unwired: 4 out]
                                }
                                n3492 = for {
                                tunnel: w4835 -> [w4844] mode=indexing
                                tunnel: [w4843] -> w4827 mode=indexing
                                n3493 = Fract/Exp String To Number(string=w4844) -> (number=w4843:dbl)  [unwired: 4 out]
                                }
                                n3494 = for {
                                tunnel: w4830 -> [w4842] mode=indexing
                                tunnel: [w4841] -> w4828 mode=indexing
                                n3495 = Fract/Exp String To Number(string=w4842) -> (number=w4841:dbl)  [unwired: 4 out]
                                }
                                n3496 = global write "读配置文件全局2.vi" "一级故障阀值"(w4826) -> ()
                                n3497 = global write "读配置文件全局2.vi" "二级故障阀值"(w4827) -> ()
                                n3498 = global write "读配置文件全局2.vi" "三级故障阀值"(w4828) -> ()
                              }
                              frame #2 {
                                n3499 = Index Array(array=w4883, index (col)=5 ("禁用的索引 (列)")) -> (element=w4881:string[])  [unwired: 1 in]
                                n3500 = Delete From Array(array=w4881, length=1 ("长度"), index=16 ("索引")) -> (deleted portion=w4877:string[], array with subset deleted=w4878:string[])
                                n3501 = for {
                                tunnel: w4878 -> [w4886] mode=indexing
                                tunnel: [w4885] -> w4882 mode=indexing
                                n3502 = Fract/Exp String To Number(string=w4886) -> (number=w4885:dbl)  [unwired: 4 out]
                                }
                                n3503 = Index Array(array=w4882) -> (element #1=w4876:dbl, element #2=w4875:dbl, element #3=w4874:dbl, element #4=w4873:dbl, element #5=w4872:dbl, element #6=w4871:dbl, element #7=w4870:dbl, element #8=w4869:dbl, element #9=w4868:dbl, element #10=w4867:dbl, element #11=w4866:dbl, element #12=w4857:dbl, element #13=w4865:dbl, element #14=w4864:dbl, element #15=w4863:dbl, element #16=w4862:dbl, element #17=w4855:dbl, element #18=w4854:dbl, element #19=w4853:dbl, element #20=w4852:dbl, element #21=w4851:dbl, element #22=w4850:dbl)  [unwired: 22 in]
                                n3504 = Build Array("配置文件读取完成") -> (w4860:string[])
                                n3505 = Index Array(array=w4877, index=22 ("索引")) -> (element=w4856:string)
                                n3506 = global read "读配置文件全局2.vi" "电池组信息"() -> (w4848:T29)
                                n3507 = call "表格编辑.vi"("新元素/子数组"=w4860, "活动单元格:单元格背景色"=u32 6618880, "MCListbox引用句柄"=w4859) -> ()  [unwired: 9 out]
                                n3508 = Bundle(cluster=w4848, "电池类型"=w4876, "电池厂家"=w4875, "电池地区"=w4874, "电池组序号"=w4873, "电池包串联数"=w4872, "电池包并联数"=w4871, "电池包安时数"=w4870, "电池包序号"=w4869, "充电次数"=w4868, "充满电时间"=w4867, "放空时间"=w4866, "车牌号"=w4856, "最大允许单体电压"=w4857, "最大允许总电压"=w4865, "最大允许温度"=w4864, "最小允许温度"=w4863, "最大允许充电电流"=w4862, "最小允许充电电流"=w4855, "最小允许单体电压"=w4854, "电流步长"=w4853, "SOC"=w4852, "充电总安时"=w4851, "放电总这时"=w4850) -> (w4847:T29)
                                n3509 = call <vilib>:"Unset Busy.vi"() -> ()  [unwired: 2 in, 10 out]
                                n3510 = global write "读配置文件全局2.vi" "电池组信息"(w4847) -> ()
                              }
                            }
                          }
                        }
                      }
                      frame True {
                      }
                    }
                  }
                  frame Enabled {
                  }
                }
                n3511 = case shown="\"从板\"" w4698 {
                  frame "主板", Default {
                    w4887 = FALSE
                    n3512 = global write "读配置文件全局.vi" "SOC判定"(w4887) -> ()
                    n3513 = global write "读配置文件全局.vi" "SOH判定"(w4887) -> ()
                    n3514 = global write "读配置文件全局.vi" "车牌号判定"(w4887) -> ()
                    n3515 = global write "读配置文件全局.vi" "电池信息1判定"(w4887) -> ()
                    n3516 = global write "读配置文件全局.vi" "保险位置判定"(w4887) -> ()
                    n3517 = global write "读配置文件全局.vi" "产品编号判定"(w4887) -> ()
                    n3518 = global write "读配置文件全局.vi" "充放电安时判定"(w4887) -> ()
                    n3519 = global write "读配置文件全局.vi" "从板个数判定"(w4887) -> ()
                    n3520 = global write "读配置文件全局.vi" "电池包组号判定"(w4887) -> ()
                    n3521 = global write "读配置文件全局.vi" "电压个数判定"(w4887) -> ()
                    n3522 = global write "读配置文件全局.vi" "电压起始值判定"(w4887) -> ()
                    n3523 = global write "读配置文件全局.vi" "二级故障判定"(w4887) -> ()
                    n3524 = global write "读配置文件全局.vi" "三级故障判定"(w4887) -> ()
                    n3525 = global write "读配置文件全局.vi" "通道电压数判定"(w4887) -> ()
                    n3526 = global write "读配置文件全局.vi" "温度个数判定"(w4887) -> ()
                    n3527 = global write "读配置文件全局.vi" "一级故障判定"(w4887) -> ()
                    n3528 = global write "读配置文件全局.vi" "温度起始值判定"(w4887) -> ()
                    n3529 = global write "读配置文件全局.vi" "充电控制参数判定"(w4887) -> ()
                    n3530 = global write "读配置文件全局.vi" "电池充放电次数判定"(w4887) -> ()
                    n3531 = global write "读配置文件全局.vi" "加热控制参数判定"(w4887) -> ()
                    n3532 = global write "读配置文件全局.vi" "配置文件版本判定"(w4887) -> ()
                    n3533 = global write "读配置文件全局.vi" "电池额定实际容量判定"(w4887) -> ()
                  }
                  frame "从板" {
                    w4888 = FALSE
                    n3534 = disable-structure shown="禁用" {
                      frame Disabled {
                        n3535 = global read "读配置文件全局2.vi" "充电次数时间判定"() -> ()  [unwired: 1 in]
                        n3536 = global read "读配置文件全局2.vi" "电池包信息1判定"() -> ()  [unwired: 1 in]
                        n3537 = global read "读配置文件全局2.vi" "电池包序号判定"() -> ()  [unwired: 1 in]
                        n3538 = global read "读配置文件全局2.vi" "充放电安时判定"() -> ()  [unwired: 1 in]
                        n3539 = global read "读配置文件全局2.vi" "车牌号判定"() -> ()  [unwired: 1 in]
                        n3540 = global read "读配置文件全局2.vi" "充电参数判定"() -> ()  [unwired: 1 in]
                        n3541 = global read "读配置文件全局2.vi" "保险位置判定"() -> ()  [unwired: 1 in]
                      }
